vi "Write Active Plot.vi"(8 "error in (no error)":errorcluster, 10 "Active Plot":i32, 11 "2D Error Bar.lvclass in":refnum<class "2D Error Bar.lvclass">) -> (0 "error out":errorcluster, 3 "2D Error Bar.lvclass out":refnum<class "2D Error Bar.lvclass">)   [LabVIEW 2020, in "2D Error Bar.lvclass"]
uses:
  <vilib>/Math Plots/2D Math Plots/2D Error Bar/2D Error Bar/2D Error Bar.lvclass
  <vilib>/Math Plots/2D Math Plots/2D Error Bar/2D Error Bar/2D Error Bar.lvclass/2D Error Bar.ctl
  <vilib>/Math Plots/2D Math Plots/2D Error Bar/2D Error Bar/Typedef/2D Error Bar Property.ctl
  <vilib>/Math Plots/2D Math Plots/2D Plot/2D Plot/2D Plot.lvclass
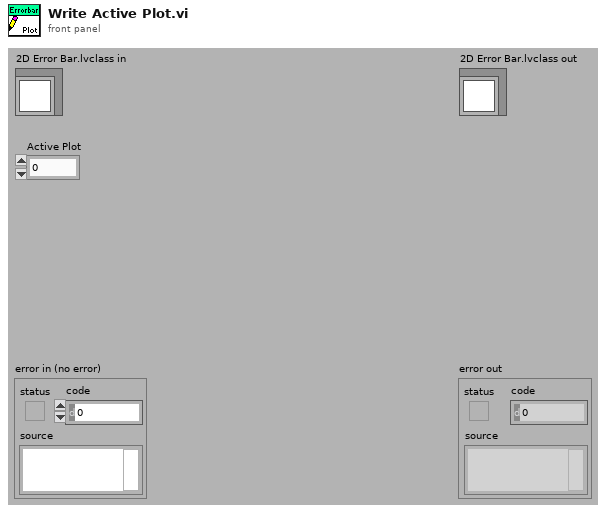
[diagram p1: front panel]
types:
  T1 = typedef "2D Error Bar.lvclass/2D Error Bar Property.ctl" = cluster{"Marker Size":dbl, "Marker Line Style":u8, "Marker Line Width":u8, "Marker Color":u32, "Error Bar Interpolation":enum16{"Show Point", "Show Line", "Show Bar"}, "Error Mode":enum16{"Show Y Error", "Show X Error", "Show Both Error"}}
  T2 = typedef "2D Plot.lvclass/Plot Property Array.ctl" = T3[]
  T3 = typedef "2D Plot.lvclass/Plot Property.ctl" = cluster{"Bar Plot Style":u8, "DigitalLineStyle":u8, "TransitionLocation":u8, "Transition Type":u8, "Fill To":i16, "Fill/Pt. Color":u32, "Label Style":u8, "Line Style":u8, "Line Width":u8, "Plot Color":u32, "Plot Interpolation":u8, "Plot Name":string, "Point Style":u8, "Visible?":bool, "XScaleIdx":u32, "YScaleIdx":u32}
  T4 = typedef "2D Error Bar.lvclass/2D Error Bar Property Array.ctl" = T1[]
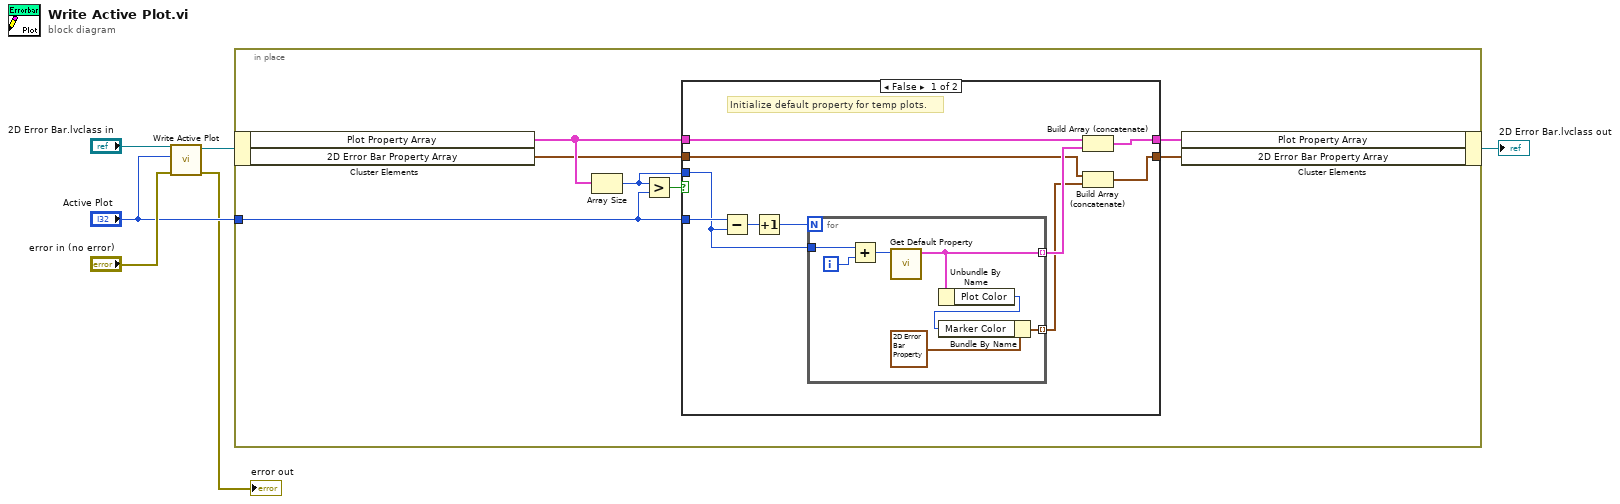
[diagram p0: block diagram]
diagram:
  n1 = call-parent "Write Active Plot.vi"("error in (no error)"="error in (no error)", "Active Plot"="Active Plot", "2D Plot.lvclass in"="2D Error Bar.lvclass in") -> ("error out"=→"error out":errorcluster, "2D Plot.lvclass out"=w3:refnum<class "2D Error Bar.lvclass">)  [unwired: 7 in]
  n2 = in-place {
    in-place-border: "Active Plot" -> [w11]
    n3 = in-place-cluster #1(w3) -> ("Plot Property Array"=w12:T2, "2D Error Bar Property Array"=w8:T4)
    n4 = Array Size(array=w12) -> (size(s)=w10:i32)
    n5 = Greater?(x=w10, y=w11) -> (0:w13:bool)
    n6 = case shown="False" w13 {
      tunnel: [w21 w32] -> w9
      tunnel: w12 -> [w23 w32]
      tunnel: w10 -> [w18 _]
      tunnel: w11 -> [w19 _]
      tunnel: w8 -> [w17 w31]
      tunnel: [w16 w31] -> w7
      frame False {
        # "Initialize default property for temp plots."
        n7 = Subtract(x=w19, y=w18) -> (x-y=w20:i32)
        n8 = Increment(x=w20) -> (x+1=w15:i32)
        n9 = for {
          N: w15 -> [_]
          tunnel: w18 -> [w29]
          tunnel: [w25] -> w22 mode=indexing
          tunnel: [w26] -> w14 mode=indexing
          i -> [w30]
          n10 = Add(x=w29, y=w30) -> (x+y=w28:i32)
          n11 = call <vilib>:"Get Default Property.vi"("Index"=w28) -> ("Temporary Property"=w25:T3)  [unwired: 10 in]
          n12 = Unbundle By Name(w25) -> ("Plot Color"=w24:u32)
          n13 = Bundle By Name(cluster=T1 {"Marker Size"=0.0, "Marker Line Style"=0, "Marker Line Width"=0, "Marker Color"=0, "Error Bar Interpolation"=enum."Show Point", "Error Mode"=enum."Show Y Error"} ("2D Error Bar Property"), "Marker Color"=w24) -> (w26:T1)
        }
        n14 = Build Array (concatenate)(w23, w22) -> (w21:T2)
        n15 = Build Array (concatenate)(w17, w14) -> (w16:T4)
      }
      frame True {
      }
    }
    n16 = in-place-cluster #1("Plot Property Array"=w9, "2D Error Bar Property Array"=w7) -> (→"2D Error Bar.lvclass out":refnum<class "2D Error Bar.lvclass">)
  }
